vi "ma_Spectrum Averaging (2ch) no State.vi"(0 "Sx":cdb[](array[numeric]), 1 "Sy":cdb[](array[numeric]), 2 "Sxx":dbl[](array[numeric]), 3 "Syy":dbl[](array[numeric]), 4 "Sxy":cdb[](array[numeric]), 5 "df":dbl format="%0.2p", 6 "retrieve last spectrum (F)":bool, 7 "averaging parameters":T3={"averaging mode"=enum."No averaging", "weighting mode"=enum."Exponential", "number of averages"=10} {"number of averages" min=1}, 8 "restart averaging (F)":bool, 9 "state info":T1 {"Syy" format="%0.2f"; "Sxy" format="%0.2f"; "Sy" format="%0.2f"; "Sxx" format="%0.2f"; "avgs completed" format="%0.2f"; "df" format="%0.2f"; "Sx" format="%0.2f"; "spectrum parameters"."window" items=["Rectangle"=0, "Hanning"=1, "Hamming"=2, "Blackman-Harris"=3, "Exact Blackman"=4, "Blackman"=5, "Flat Top"=6, "4 Term B-Harris "=7, "7 Term B-Harris"=8, "Low Sidelobe"=9, "Blackman Nuttall"=11, "Triangle"=30, "Bartlett-Hanning"=31, "Bohman"=32, "Parzen"=33, "Welch"=34, "Kaiser"=60, "Dolph-Chebyshev"=61, "Gaussian"=62]; "dt" format="%0.2f"; "timestamp" format="%0.2f"; "dt history" format="%0.2f"; "t0 history" format="%0.2f"}) -> (11 "state info out":T1 {"Syy" format="%0.2f"; "Sxy" format="%0.2f"; "Sy" format="%0.2f"; "Sxx" format="%0.2f"; "avgs completed" format="%0.2f"; "df" format="%0.2f"; "Sx" format="%0.2f"; "spectrum parameters"."window" items=["Rectangle"=0, "Hanning"=1, "Hamming"=2, "Blackman-Harris"=3, "Exact Blackman"=4, "Blackman"=5, "Flat Top"=6, "4 Term B-Harris "=7, "7 Term B-Harris"=8, "Low Sidelobe"=9, "Blackman Nuttall"=11, "Triangle"=30, "Bartlett-Hanning"=31, "Bohman"=32, "Parzen"=33, "Welch"=34, "Kaiser"=60, "Dolph-Chebyshev"=61, "Gaussian"=62]; "dt" format="%0.2f"; "timestamp" format="%0.2f"; "dt history" format="%0.2f"; "t0 history" format="%0.2f"}, 12 "df":dbl format="%0.2p", 13 "averages completed":dbl format="%0.2f", 14 "avg Sx":cdb[](array[numeric]), 15 "avg Sy":cdb[](array[numeric]), 16 "avg Sxx":dbl[](array[numeric]), 17 "avg Syy":dbl[](array[numeric]), 18 "avg Sxy":cdb[](array[numeric]), 19 "averaging done":bool)   [LabVIEW 2020, in "NI_MAPro.lvlib"]
uses:
  NI_MAPro.lvlib
  2-chan State.ctl
  windowTd.ctl
  NI_AALPro.lvlib
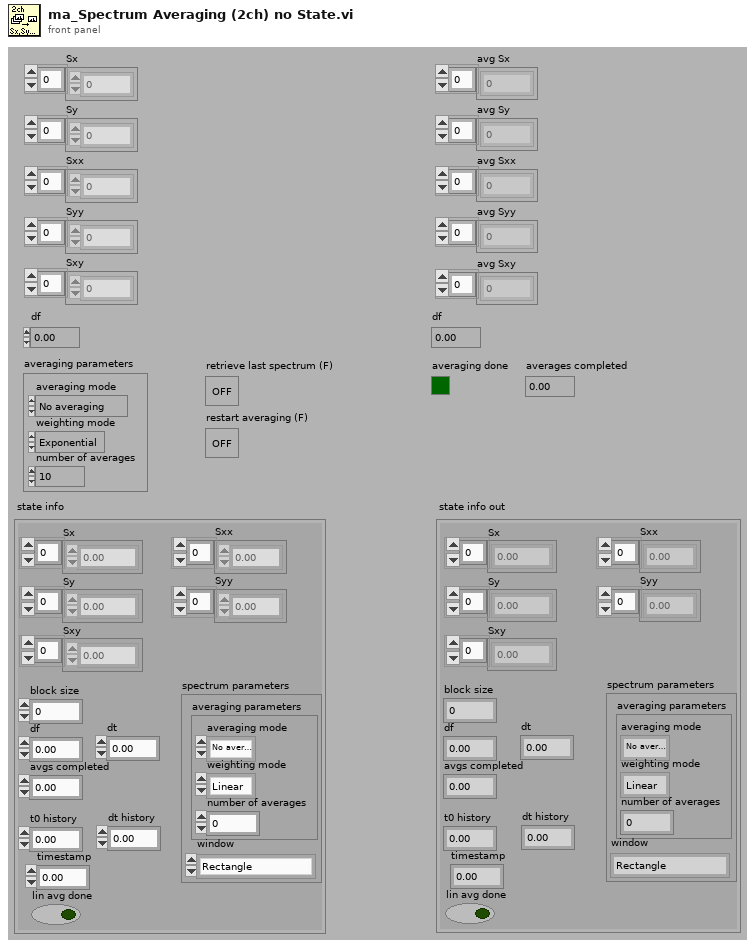
[diagram p1: front panel]
types:
  T1 = typedef "NI_MAPro.lvlib/2-chan State.ctl" = cluster{"Sx":cdb[], "Sy":cdb[], "Sxx":dbl[], "Syy":dbl[], "Sxy":cdb[], "block size":i32, "df":dbl, "dt":dbl, "avgs completed":dbl, "spectrum parameters":cluster{"averaging parameters":cluster{"averaging mode":enum16{"No averaging", "Vector averaging", "RMS averaging", "Peak hold"}, "weighting mode":enum16{"Linear", "Exponential"}, "number of averages":u32}, "window":T2}, "lin avg done":bool, "t0 history":dbl, "dt history":dbl, "timestamp":dbl}
  T2 = typedef "NI_AALPro.lvlib/windowTd.ctl" = u32
  T3 = cluster{"averaging mode":enum16{"No averaging", "Vector averaging", "RMS averaging", "Peak hold"}, "weighting mode":enum16{"Linear", "Exponential"}, "number of averages":u32}
  T4 = enum16{"No averaging", "Vector averaging", "RMS averaging", "Peak hold"}
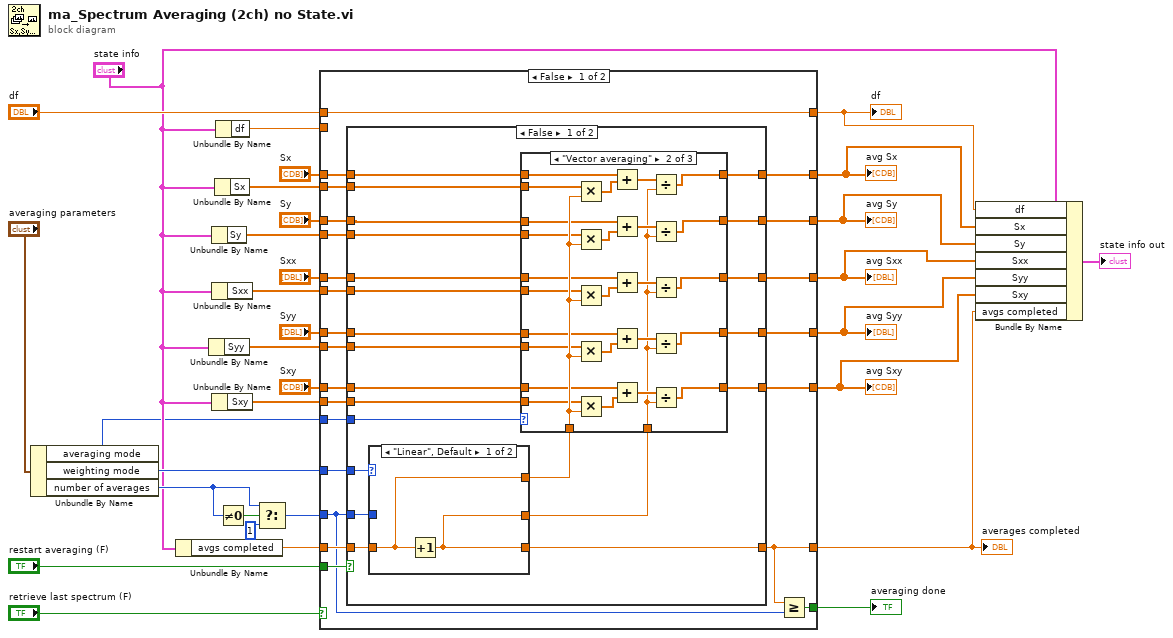
[diagram p0: block diagram]
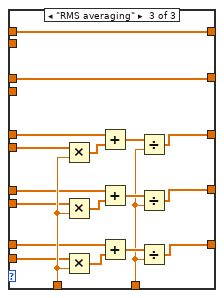
[diagram p3: hidden frame]
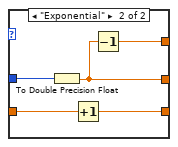
[diagram p4: hidden frame]
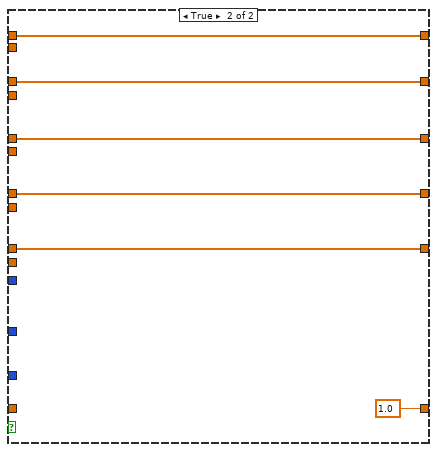
[diagram p5: hidden frame]
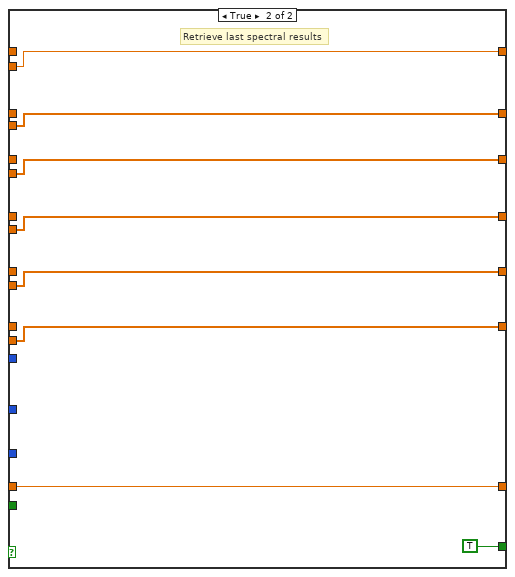
[diagram p6: hidden frame]
diagram:
  n1 = Unbundle By Name("averaging parameters") -> ("averaging mode"=w1:T4, "weighting mode"=w30:enum16{"Linear", "Exponential"}, "number of averages"=w25:u32)
  n2 = Unbundle By Name("state info") -> ("avgs completed"=w21:dbl)
  n3 = Unbundle By Name("state info") -> ("Syy"=w13:dbl[])
  n4 = Unbundle By Name("state info") -> ("Sy"=w15:cdb[])
  n5 = Unbundle By Name("state info") -> ("Sxx"=w14:dbl[])
  n6 = Unbundle By Name("state info") -> ("Sxy"=w12:cdb[])
  n7 = Unbundle By Name("state info") -> ("Sx"=w22:cdb[])
  n8 = Unbundle By Name("state info") -> ("df"=w17:dbl)
  n9 = Not Equal To 0?(x=w25) -> (x != 0?=w26:bool)
  n10 = Select(t=w25, s=w26, f=u32 1) -> (s? t:f=w23:u32)
  n11 = case shown="False" "retrieve last spectrum (F)" {
    tunnel: [w55 w149] -> w6
    tunnel: w21 -> [w54 w148]
    tunnel: w22 -> [w53 w149]
    tunnel: w30 -> [w52 _]
    tunnel: "Sx" -> [w51 _]
    tunnel: "restart averaging (F)" -> [w50 _]
    tunnel: w23 -> [w49 _]
    tunnel: [w48 w148] -> w7
    tunnel: [w47 TRUE] -> w29
    tunnel: "df" -> [w46 _]
    tunnel: [w46 w146] -> w20
    tunnel: w17 -> [_ w146]
    tunnel: w15 -> [w37 w145]
    tunnel: w14 -> [w36 w144]
    tunnel: w13 -> [w35 w143]
    tunnel: w12 -> [w34 w142]
    tunnel: "Sxy" -> [w38 _]
    tunnel: "Syy" -> [w40 _]
    tunnel: "Sxx" -> [w42 _]
    tunnel: "Sy" -> [w44 _]
    tunnel: [w45 w145] -> w5
    tunnel: [w43 w144] -> w2
    tunnel: [w41 w143] -> w4
    tunnel: [w39 w142] -> w3
    tunnel: w1 -> [w33 _]
    frame False {
      n12 = case shown="False" w50 {
        tunnel: [w76 w140] -> w55
        tunnel: [w72 1.0] -> w48
        tunnel: w54 -> [w74 _]
        tunnel: w53 -> [w77 _]
        tunnel: w51 -> [w75 w140]
        tunnel: w52 -> [w73 _]
        tunnel: w49 -> [w71 _]
        tunnel: [w68 w139] -> w45
        tunnel: w44 -> [w67 w139]
        tunnel: [w59 w138] -> w43
        tunnel: w42 -> [w66 w138]
        tunnel: [w57 w137] -> w41
        tunnel: w40 -> [w65 w137]
        tunnel: [w58 w136] -> w39
        tunnel: w38 -> [w64 w136]
        tunnel: w37 -> [w63 _]
        tunnel: w36 -> [w62 _]
        tunnel: w35 -> [w61 _]
        tunnel: w34 -> [w60 _]
        tunnel: w33 -> [w56 _]
        frame False {
          n13 = case shown="\"Linear\", Default" w73 {
            tunnel: w74 -> [w129 w134]
            tunnel: [w130 w135] -> w72
            tunnel: [w129 w131] -> w70
            tunnel: [w130 w132] -> w69
            tunnel: w71 -> [_ w133]
            frame "Linear", Default {
              n14 = Increment(x=w129) -> (x+1=w130:dbl)
            }
            frame "Exponential" {
              n15 = To Double Precision Float(number=w133) -> (double precision float=w132:dbl)
              n16 = Increment(x=w134) -> (x+1=w135:dbl)
              n17 = Decrement(x=w132) -> (x-1=w131:dbl)
            }
          }
          n18 = case shown="\"Vector averaging\"" w56 {
            tunnel: w77 -> [_ w109 _]
            tunnel: [w82 w107 w111] -> w76
            tunnel: w75 -> [w82 w106 w111]
            tunnel: w70 -> [_ w96 w122]
            tunnel: w69 -> [_ w95 w121]
            tunnel: [w81 w94 w110] -> w68
            tunnel: w67 -> [w81 w93 w110]
            tunnel: w66 -> [w80 w92 w120]
            tunnel: w65 -> [w79 w91 w119]
            tunnel: w64 -> [w78 w90 w118]
            tunnel: w63 -> [_ w89 _]
            tunnel: w62 -> [_ w88 w117]
            tunnel: w61 -> [_ w87 w116]
            tunnel: w60 -> [_ w86 w115]
            tunnel: [w80 w85 w114] -> w59
            tunnel: [w78 w84 w113] -> w58
            tunnel: [w79 w83 w112] -> w57
            frame "No averaging", Default {
            }
            frame "Vector averaging" {
              n19 = Multiply(x=w109, y=w96) -> (x*y=w108:cdb[])
              n20 = Multiply(x=w89, y=w96) -> (x*y=w103:cdb[])
              n21 = Multiply(x=w88, y=w96) -> (x*y=w102:dbl[])
              n22 = Multiply(x=w87, y=w96) -> (x*y=w99:dbl[])
              n23 = Multiply(x=w86, y=w96) -> (x*y=w98:cdb[])
              n24 = Add(x=w106, y=w108) -> (x+y=w105:cdb[])
              n25 = Add(x=w93, y=w103) -> (x+y=w104:cdb[])
              n26 = Add(x=w92, y=w102) -> (x+y=w101:dbl[])
              n27 = Add(x=w91, y=w99) -> (x+y=w100:dbl[])
              n28 = Add(x=w90, y=w98) -> (x+y=w97:cdb[])
              n29 = Divide(x=w105, y=w95) -> (x/y=w107:cdb[])
              n30 = Divide(x=w104, y=w95) -> (x/y=w94:cdb[])
              n31 = Divide(x=w101, y=w95) -> (x/y=w85:dbl[])
              n32 = Divide(x=w100, y=w95) -> (x/y=w83:dbl[])
              n33 = Divide(x=w97, y=w95) -> (x/y=w84:cdb[])
            }
            frame "RMS averaging" {
              n34 = Multiply(x=w117, y=w122) -> (x*y=w128:dbl[])
              n35 = Multiply(x=w116, y=w122) -> (x*y=w125:dbl[])
              n36 = Multiply(x=w115, y=w122) -> (x*y=w124:cdb[])
              n37 = Add(x=w120, y=w128) -> (x+y=w127:dbl[])
              n38 = Add(x=w119, y=w125) -> (x+y=w126:dbl[])
              n39 = Add(x=w118, y=w124) -> (x+y=w123:cdb[])
              n40 = Divide(x=w127, y=w121) -> (x/y=w114:dbl[])
              n41 = Divide(x=w126, y=w121) -> (x/y=w112:dbl[])
              n42 = Divide(x=w123, y=w121) -> (x/y=w113:cdb[])
            }
          }
        }
        frame True {
        }
      }
      n43 = Greater Or Equal?(x=w48, y=w49) -> (x >= y?=w47:bool)
    }
    frame True {
      # "Retrieve last spectral results"
    }
  }
  "avg Sxy" <- w3
  "averages completed" <- w7
  "averaging done" <- w29
  "df" <- w20
  "avg Sxx" <- w2
  "avg Syy" <- w4
  "avg Sy" <- w5
  "avg Sx" <- w6
  n44 = Bundle By Name(cluster="state info", "df"=w20, "Sx"=w6, "Sy"=w5, "Sxx"=w2, "Syy"=w4, "Sxy"=w3, "avgs completed"=w7) -> (→"state info out":T1)
